vi "Dispose Log Service.vi"(8 "error in (no error)":errorcluster, 11 "Log Service in":refnum<data-value>) -> (0 "error out":errorcluster)   [LabVIEW 2019, in "Utility API.lvlib" / "Log Service.lvclass"]
doc: "<b>Description</b> Dispose log service"
uses:
  Log Service.lvclass
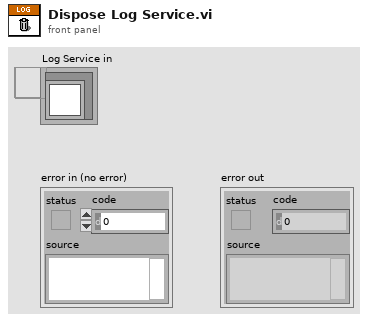
[diagram p1: front panel]
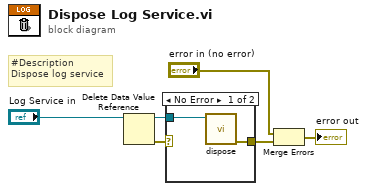
[diagram p0: block diagram]
diagram:
  # "#Description\nDispose log service"
  n1 = Delete Data Value Reference(data value reference="Log Service in") -> (data value=w3:refnum<class "Log Service.lvclass">, error out=w2:errorcluster)  [unwired: 1 in]
  n2 = case shown="No Error" w2 {
    selector: w2 -> [_ w9]
    tunnel: w3 -> [w8 _]
    tunnel: [w7 w9] -> w1
    frame No Error {
      n3 = call-dynamic "dispose.vi"("Log Service in"=w8) -> ("error out"=w7:errorcluster)  [unwired: 10 in]
    }
    frame Error {
    }
  }
  n4 = Merge Errors("error in (no error)", w1) -> (→"error out":errorcluster)
